vi "Check_Invalid_Characters_In_Name.vi"(6 "AB_Destination in":refnum<class "AB_Destination.lvclass">, 7 "AB_Source in":refnum<class "AB_Source.lvclass">, 8 "error in (no error)":errorcluster, 9 "update name":bool, 10 "file name in":string, 11 "Build in":refnum<class "AB_Build.lvclass">) -> (0 "error out":errorcluster, 1 "updated":bool, 2 "file name out":string, 3 "Build out":refnum<class "AB_Build.lvclass">, 5 "AB_Source out":refnum<class "AB_Source.lvclass">)   [LabVIEW 2020, in "AB_Build.lvclass"]
uses:
  <vilib>/AppBuilder/AB_Classes/Build/AB_Build.lvclass
  <vilib>/AppBuilder/AB_Classes/Destination/AB_Destination.lvclass
  <vilib>/AppBuilder/AB_Classes/Source/AB_Source.lvclass
  <resource>/Framework/Providers/Common/provcom_StringGlobals.vi
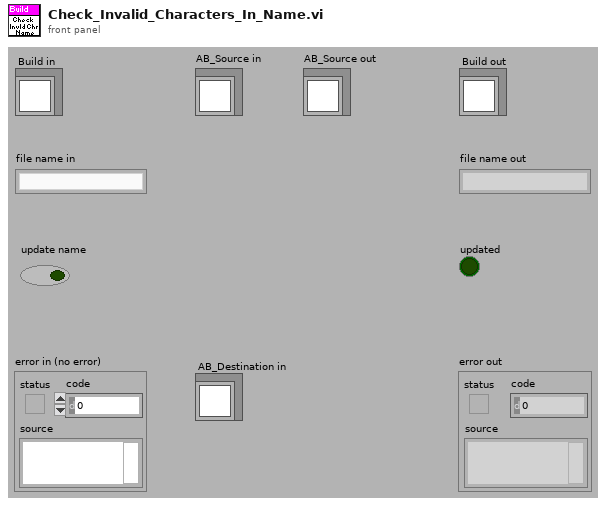
[diagram p1: front panel]
types:
  T1 = enum32{"invalid OS target", "Mac OS", "Windows 3.1", "Windows 95/NT", "Solaris 1", "Solaris 2", "HP-UX", "PowerMAX", "Linux", "Irix", "Rhapsody", "BeOS", "AIX", "OSF1", "VxWorks", "PharLap", "Carbon", "RTX", "Windows x64", "Linux x64", "Mac OS X x64"}
  T2 = typedef "AB_Source.ctl" = cluster{"path":path, "itemID":string, "parentIndex":i32, "sourceInclusion":T3, "destinationIndex":i32, "properties":T4[], "newName":string, "lvfile":bool, "valid":bool, "eng_inBuild":bool, "eng_isNonVILink":bool, "Amalgamation":bool, "Amalgamation Piece":bool, "eng_delimitedName":string, "preventRename":bool}
  T3 = typedef "AB_Source_Inclusion.ctl" = enum16{"IncludeIfReferenced", "Include", "Exclude", "TopLevel"}
  T4 = typedef "AB_Source_Properties.ctl" = cluster{"sourcePropertyType":T5, "value":variant}
  T5 = typedef "AB_Source_Property_Type.ctl" = enum16{"Remove block diagram", "Remove front panel", "Password", "Window has title bar", "Show menu bar", "Show vertical scroll bar", "Show horizontal scroll bar", "Show toolbar", "Show Abort button", "Show fp when called", "Window behavior", "Allow user to close window", "Window run-time position", "Run when opened", "Allow debugging", "Auto error handling", "Generate guard code", "Use stack variables", "Expression folding", "Integer only", "Inline subVI"}
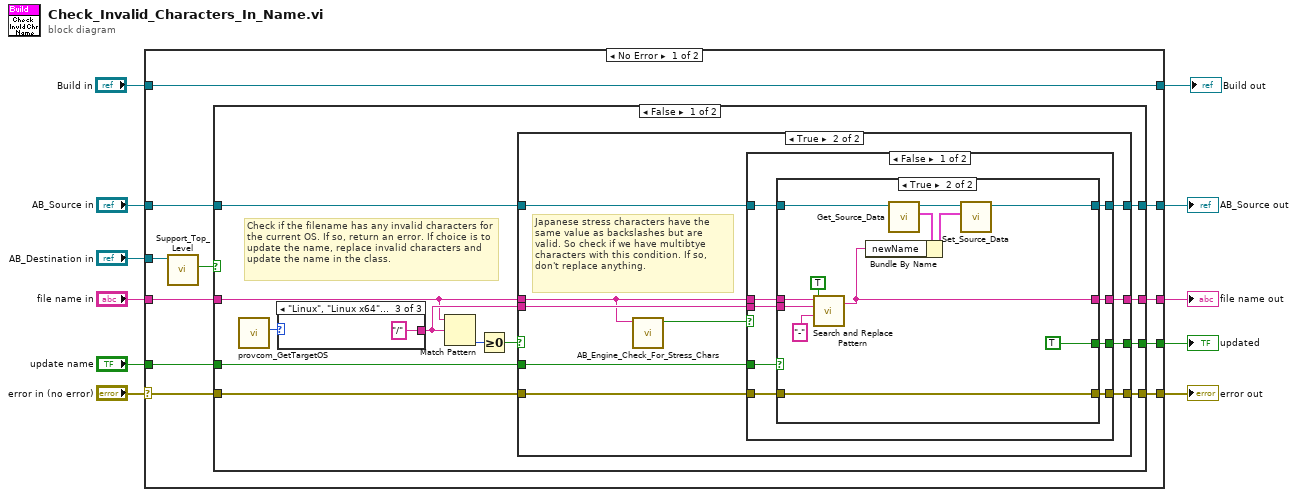
[diagram p0: block diagram]
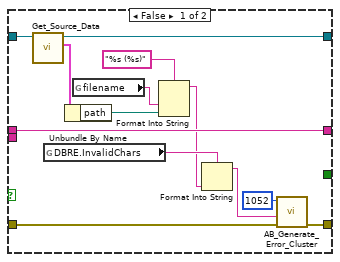
[diagram p3: hidden frame]
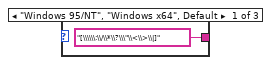
[diagram p5: hidden frame]
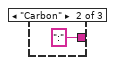
[diagram p6: hidden frame]
diagram:
  n1 = case shown="No Error" "error in (no error)" {
    selector: "error in (no error)" -> [w16 w93]
    tunnel: [w15 w93] -> w10
    tunnel: [w22 w92] -> w8
    tunnel: "Build in" -> [w22 w92]
    tunnel: "AB_Destination in" -> [w21 _]
    tunnel: "file name in" -> [w19 _]
    tunnel: [w18 _] -> w5
    tunnel: "AB_Source in" -> [w17 w91]
    tunnel: "update name" -> [w14 _]
    tunnel: [w13 w91] -> w2
    tunnel: [w12 _] -> w1
    frame No Error {
      n2 = call-dynamic "Support_Top_Level.vi"("AB_Destination in"=w21) -> ("supportTopLevel"=w20:bool)  [unwired: 1 in, 9 out]
      n3 = case shown="False" w20 {
        tunnel: w19 -> [w29 w90]
        tunnel: [w30 w90] -> w18
        tunnel: w17 -> [w28 w88]
        tunnel: w16 -> [w27 w89]
        tunnel: [w25 w89] -> w15
        tunnel: w14 -> [w26 _]
        tunnel: [w24 w88] -> w13
        tunnel: [w23 _] -> w12
        frame False {
          # "Check if the filename has any invalid characters for the current OS. If so, return an error. If choice is to update the name, replace invalid characters and update the name in the class."
          n4 = call <resource>:"provcom_GetTargetOS.vi"() -> ("App.TargetOS"=w34:T1)  [unwired: 11 out]
          n5 = case shown="\"Linux\", \"Linux x64\", \"Mac OS X x64\"" w34 {
            tunnel: ["[\\\\\\:\\/\\*\\?\\\"\\<\\>\\|]" ":" "/"] -> w31
            frame "Windows 95/NT", "Windows x64", Default {
            }
            frame "Carbon" {
            }
            frame "Linux", "Linux x64", "Mac OS X x64" {
            }
          }
          n6 = Match Pattern(string=w29, regular expression=w31) -> (offset past match=w33:i32)  [unwired: 4 out]
          n7 = Greater Or Equal To 0?(x=w33) -> (x >= 0?=w32:bool)
          n8 = case shown="True" w32 {
            tunnel: w29 -> [w37 w39]
            tunnel: [w37 w47] -> w30
            tunnel: w31 -> [_ w46]
            tunnel: w28 -> [w35 w42]
            tunnel: w27 -> [w36 w45]
            tunnel: w26 -> [_ w44]
            tunnel: [w36 w43] -> w25
            tunnel: [w35 w41] -> w24
            tunnel: [_ w40] -> w23
            frame False {
            }
            frame True {
              # "Japanese stress characters have the same value as backslashes but are valid. So check if we have multibtye characters with this condition. If so, don't replace anything."
              n9 = call <vilib>:"AB_Engine_Check_For_Stress_Chars.vi"("string"=w39) -> ("has stress chars"=w38:bool)  [unwired: 9 in, 1 out]
              n10 = case shown="False" w38 {
                tunnel: [w56 w83] -> w47
                tunnel: w46 -> [w55 _]
                tunnel: w45 -> [w54 w82]
                tunnel: w44 -> [w53 _]
                tunnel: [w52 w82] -> w43
                tunnel: w42 -> [w51 w84]
                tunnel: [w50 w84] -> w41
                tunnel: [w49 _] -> w40
                tunnel: w39 -> [w48 w83]
                frame False {
                  n11 = case shown="True" w53 {
                    tunnel: w48 -> [w66 w74]
                    tunnel: [w66 w72] -> w56
                    tunnel: w55 -> [_ w73]
                    tunnel: w54 -> [w68 w81]
                    tunnel: [w67 w81] -> w52
                    tunnel: w51 -> [w65 w80]
                    tunnel: [w64 w78] -> w50
                    tunnel: [_ TRUE] -> w49
                    frame False {
                      n12 = call <vilib>:"Get_Source_Data.vi"("Class in"=w65) -> ("data"=w63:T2, "Class out"=w64:refnum<class "AB_Source.lvclass">)  [unwired: 1 in, 8 out]
                      n13 = global read "provcom_StringGlobals.vi" "DBRE.InvalidChars"() -> (w59:string)
                      n14 = Unbundle By Name(w63) -> ("path"=w61:path)
                      n15 = global read "provcom_StringGlobals.vi" "filename"() -> (w60:string)
                      n16 = Format Into String(format string="%s (%s)", w60, w61) -> (resulting string=w58:string)  [unwired: 2 in, 1 out]
                      n17 = Format Into String(format string=w59, w58) -> (resulting string=w57:string)  [unwired: 2 in, 1 out]
                      n18 = call <vilib>:"AB_Generate_Error_Cluster.vi"("error in (no error)"=w68, "Additional Message"=w57, "Code"=1052) -> ("error out"=w67:errorcluster)  [unwired: 1 in, 7 out]
                    }
                    frame True {
                      n19 = call <vilib>:"Search and Replace Pattern.vi"("string"=w74, "regular expression (\"\")"=w73, "replace string (\"\")"="-" ("replace string (\"\")"), "replace all? (F)"=TRUE) -> ("result string"=w72:string)  [unwired: 2 out]
                      n20 = call <vilib>:"Get_Source_Data.vi"("Class in"=w80) -> ("data"=w77:T2, "Class out"=w79:refnum<class "AB_Source.lvclass">)  [unwired: 1 in, 8 out]
                      n21 = Bundle By Name(cluster=w77, "newName"=w72) -> (w76:T2)
                      n22 = call <vilib>:"Set_Source_Data.vi"("data"=w76, "Class in"=w79) -> ("Class out"=w78:refnum<class "AB_Source.lvclass">)  [unwired: 1 in, 8 out]
                    }
                  }
                }
                frame True {
                }
              }
            }
          }
        }
        frame True {
          # "LLBs (which are the only dest types that support top-level) can have files with names not valid by the OS. So, skip any checks."
        }
      }
    }
    frame Error {
    }
  }
  "error out" <- w10
  "Build out" <- w8
  "file name out" <- w5
  "AB_Source out" <- w2
  "updated" <- w1
